vi "Update Dependencies from Project.vi"(8 "error in (no error)":errorcluster, 10 "lvproj Path":path, 11 "PackageAbstract in":refnum<class "PackageAbstract.lvclass">) -> (0 "error out":errorcluster, 3 "PackageAbstract out":refnum<class "PackageAbstract.lvclass">)   [LabVIEW 2020, in "GPack.lvlib" / "PackageAbstract.lvclass"]
uses:
  PackageAbstract.lvclass
  LVProject/LVProject.lvclass
  GPack.lvlib
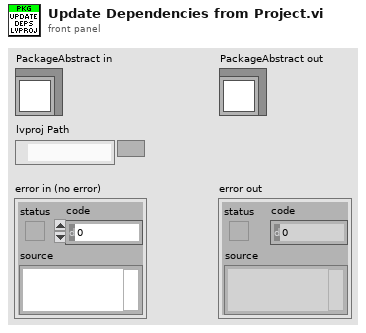
[diagram p1: front panel]
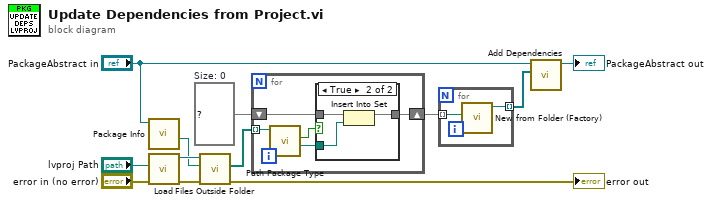
[diagram p0: block diagram]
diagram:
  w7 = set{path} {}  # Size: 0
  n1 = call-dynamic "Package Info.vi"("Package in"="PackageAbstract in") -> ("Folder"=w5:path)  [unwired: 8 in, 2 out]
  n2 = call "Load.vi"("error in (no error)"="error in (no error)", "Path"="lvproj Path") -> ("error out"=w10:errorcluster, "LVProject out"=w9:refnum<class "LVProject.lvclass">)  [unwired: 8 in]
  n3 = call "Files Outside Folder.vi"("error in (no error)"=w10, "Folder"=w5, "LVProject in"=w9) -> ("error out"=→"error out":errorcluster, "External Files"=w8:path[])  [unwired: 6 in, 1 out]
  n4 = for {
    tunnel: w8 -> [w17] mode=indexing
    shift-right: [w13] -> w4
    shift-left: w7 -> [w16]
    n5 = call "Path Package Type.vi"("Path"=w17) -> ("Root Folder"=w15:path, "Matched"=w14:bool)  [unwired: 7 in, 2 out]
    n6 = case shown="True" w14 {
      tunnel: w16 -> [w18 w21]
      tunnel: w15 -> [_ w20]
      tunnel: [w18 w19] -> w13
      frame False {
      }
      frame True {
        n7 = Insert Into Set(10:w20, 11:w21) -> (3:w19:set{path})  [unwired: 1 out]
      }
    }
  }
  n8 = for {
    tunnel: w4 -> [w23] mode=indexing
    tunnel: [w22] -> w2 mode=indexing
    n9 = call "New from Folder (Factory).vi"("Folder"=w23) -> ("PackageAbstract out"=w22:refnum<class "PackageAbstract.lvclass">)  [unwired: 9 in, 1 out]
  }
  n10 = call "Add Dependencies.vi"("Dependencies"=w2, "PackageAbstract in"="PackageAbstract in") -> ("PackageAbstract out"=→"PackageAbstract out":refnum<class "PackageAbstract.lvclass">)  [unwired: 8 in, 1 out]
